vi "Initialize.vi"(5 "Dictionary File Path":path, 11 "error in":errorcluster) -> (6 "Dictionary File Path out":path, 8 "Languages":string[](array[string]), 10 "Current Language":string, 15 "error out":errorcluster)   [LabVIEW 2017, in "JKI Simple Localization.lvlib"]
doc: "Loads the language dictionary from file.\n\nReturns the current language (defined by the OS), and available languages in the dictionary."
uses:
  JKI Simple Localization.lvlib
  Definitions/Dictionary--Cluster.ctl
  Definitions/Private/FontCluster.ctl
  Definitions/Private/Phrase Dictionary.ctl
  Definitions/Private/Translation.Action.ctl
panel:
  out "Dictionary":T1
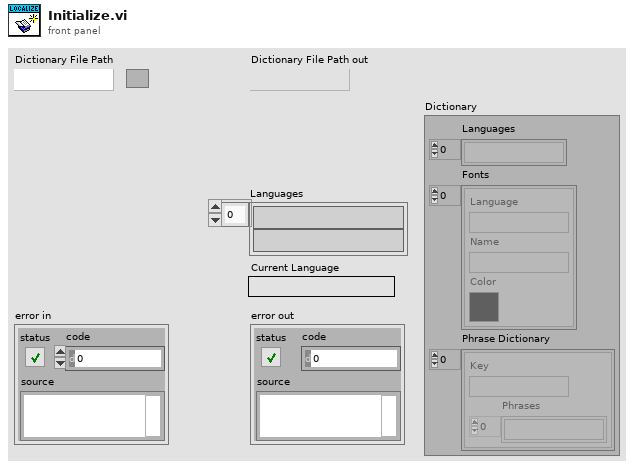
[diagram p1: front panel]
types:
  T1 = typedef "JKI Simple Localization.lvlib/Dictionary--Cluster.ctl" = cluster{"Languages":string[], "Fonts":T2[], "Phrase Dictionary":T3[]}
  T2 = typedef "JKI Simple Localization.lvlib/FontCluster.ctl" = cluster{"Language":string, "Name":string, "Color":u32}
  T3 = typedef "JKI Simple Localization.lvlib/Phrase Dictionary.ctl" = cluster{"Key":string, "Phrases":string[]}
  T4 = typedef "JKI Simple Localization.lvlib/Translation.Action.ctl" = enum16{"Read Dictionary", "Translate VIs", "Register VI", "Get Languages", "Translate Phrase", "Translate VI", "Unregister"}
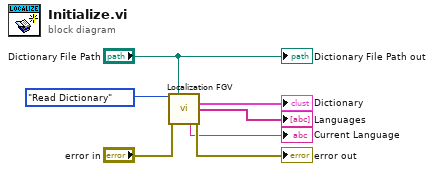
[diagram p0: block diagram]
diagram:
  n1 = call "Localization FGV.vi"("Action"=Translation.Action."Read Dictionary", "Dictionary File Path"="Dictionary File Path", "error in"="error in") -> ("Dictionary"=→"Dictionary":T1, "Languages"=→"Languages":string[], "Current Language"=→"Current Language":string, "error out"=→"error out":errorcluster)  [unwired: 8 in, 1 out]
  "Dictionary File Path out" <- "Dictionary File Path"
